vi "Display.vi"(8 "error in":errorcluster, 11 "Custom - One Button in":refnum<class "Custom - One Button.lvclass">) -> (0 "error out":errorcluster, 3 "Custom - One Button out":refnum<class "Custom - One Button.lvclass">)   [LabVIEW 2021, in "Pop-Up.lvlib" / "Custom - One Button.lvclass"]
doc: "This VI will display the custom image and message to the user\n\n<b>Code Developed By:</b> +\nDaniel Coons +\nhttps://github.com/danielcoons/tsc-pop-up"
uses:
  Custom - One Button.lvclass
  C:/Development/Open Source/tsc-pop-up/Popup/Popup.lvclass
  Popup/Popup.lvclass/Popup.ctl
  Popup/Data Member Access/Read Theme.vi
  Theme/Theme.lvclass
  Popup/Popup.lvclass
  user32.dll
panel:
  out "header":bool
  in  "OK":bool
  out "2D Picture":picture
  out "Message":string
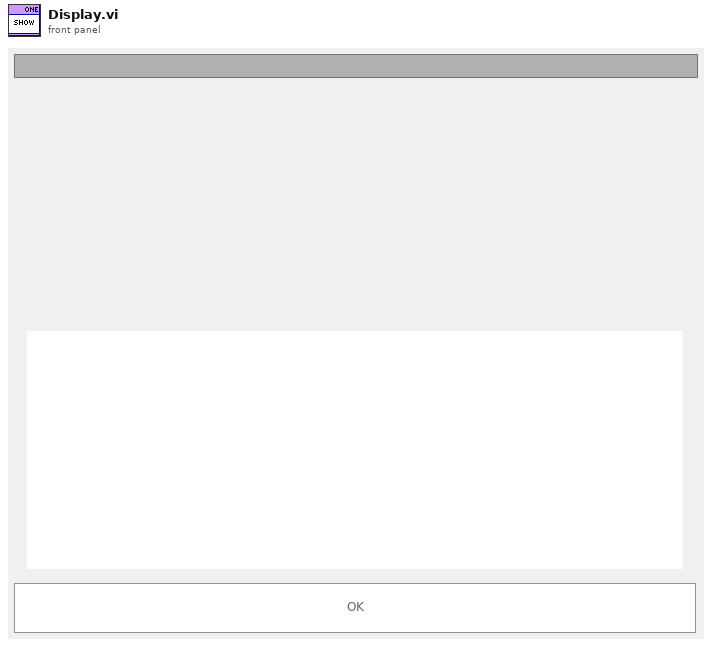
[diagram p1: front panel]
types:
  T1 = typedef "LVPoint32TypeDef.ctl" = cluster{"Horizontal":i32, "Vertical":i32}
  T2 = typedef "LVPositionTypeDef.ctl" = cluster{"Left":i32, "Top":i32}
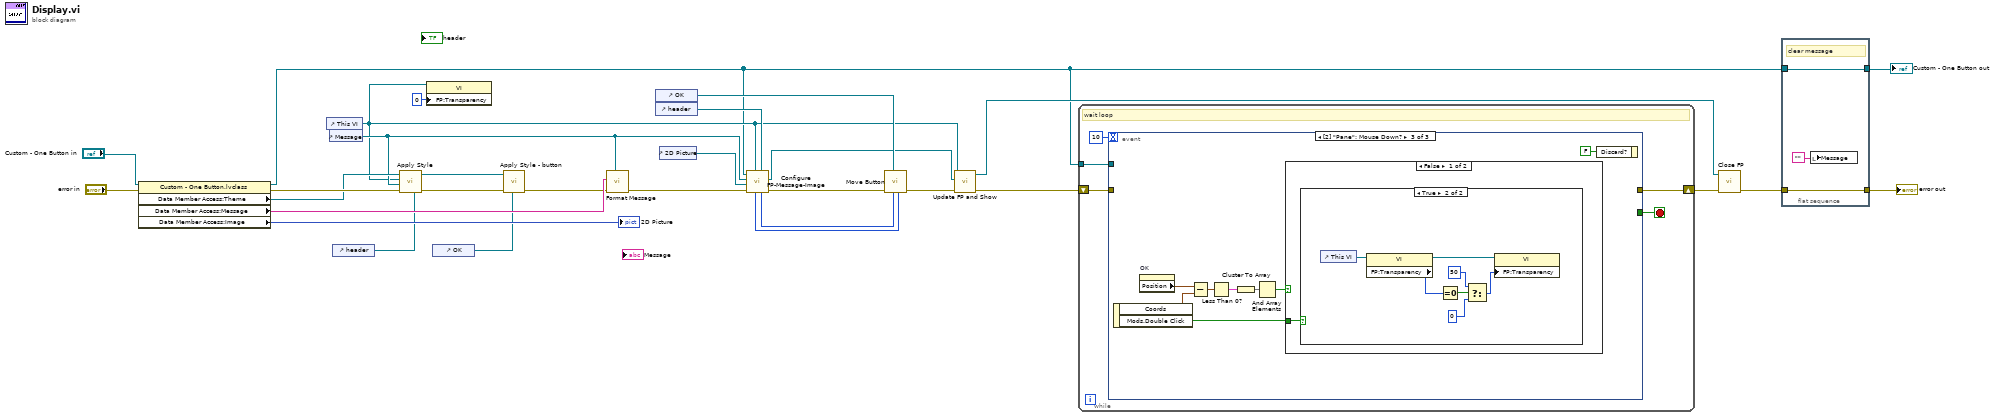
[diagram p0: block diagram]
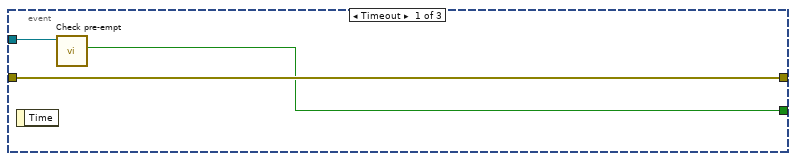
[diagram p2: hidden frame]
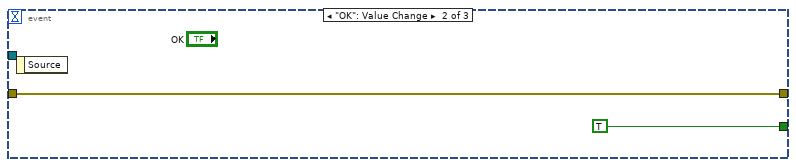
[diagram p3: hidden frame]
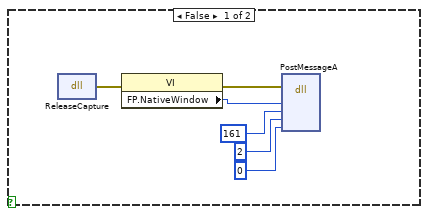
[diagram p4: hidden frame]
diagram:
  n1 = property class="Custom - One Button.lvclass"(reference="Custom - One Button in", error in="error in") -> (reference out=w1:refnum<class "Custom - One Button.lvclass">, error out=w26:errorcluster, "Data Member Access:Theme"=w21:refnum<class "Theme.lvclass">, "Data Member Access:Message"=w19:string, "Data Member Access:Image"=→"2D Picture":picture)
  n2 = control-ref of="This VI"() -> (w3:refnum<vi>)
  n3 = control-ref of="Message"() -> (w15:refnum<vi>)
  n4 = control-ref of="header"() -> (w7:refnum<vi>)
  n5 = call "Apply Style.vi"("header ref"=w7, "error in"=w26, "message ref"=w15, "pop up ref"=w3, "Theme in"=w21) -> ("error out"=w9:errorcluster, "Theme out"=w18:refnum<class "Theme.lvclass">)  [unwired: 5 in]
  n6 = property class="VI"(reference=w3, "FP:Transparency"=u8 0 ("Front Panel Window:Transparency")) -> ()  [unwired: 1 in, 2 out]
  n7 = control-ref of="OK"() -> (w17:refnum<vi>)
  n8 = call "Apply Style - button.vi"("button ref"=w17, "error in"=w9, "Theme in"=w18) -> ("error out"=w8:errorcluster)  [unwired: 7 in, 1 out]
  n9 = call "Format Message.vi"("formatted string"=w15, "error in"=w8, "String Input"=w19) -> ("error out"=w5:errorcluster)  [unwired: 7 in, 1 out]
  n10 = control-ref of="OK"() -> (w16:refnum<vi>)
  n11 = control-ref of="header"() -> (w10:refnum<vi>)
  n12 = control-ref of="2D Picture"() -> (w14:refnum<vi>)
  n13 = call "Configure FP-Message-Image.vi"("header ref"=w10, "Pop Up ref"=w3, "error in (no error)"=w5, "Image ref"=w14, "Message ref"=w15, "Popup in"=w1) -> ("error out"=w6:errorcluster, "Panel Ref"=w11:refnum<vi>, "Panel Width"=w13:i32, "Panel Height"=w12:i32)  [unwired: 1 in, 1 out]
  n14 = call "Move Button.vi"("Panel Height"=w12, "Panel Width"=w13, "Button"=w16, "error in"=w6) -> ("error out"=w25:errorcluster)  [unwired: 6 in, 1 out]
  n15 = call "Update FP and Show.vi"("error in (no error)"=w25, "Panel Ref"=w11, "VI in"=w3) -> ("error out"=w22:errorcluster, "VI out"=w4:refnum<vi>)  [unwired: 7 in]
  n16 = while {
    shift-right: [w35] -> w24
    shift-left: w22 -> [w34]
    tunnel: w1 -> [w31]
    stop <- w33 stop-if-true
    # "wait loop"
    n17 = event shown="[2] \"Pane\": Mouse Down?" {
      selector: _ -> [_ _ _]
      dyn-events: _ -> [_ _ _]
      timeout: 10 -> [_ _ _]
      tunnel: w34 -> [w38 w40 _]
      tunnel: [w38 w40 _] -> w35
      tunnel: [w36 TRUE _] -> w33
      tunnel: w31 -> [w37 _ _]
      event Timeout {
        n18 = event-data() -> ()  [unwired: 1 in, 1 out]
        n19 = call "Check pre-empt.vi"("_Popup in"=w37) -> ("Pre-empted?"=w36:bool)  [unwired: 8 in, 2 out]
      }
      event "OK": Value Change {
        n20 = event-data() -> ()  [unwired: 1 in, 1 out]
      }
      event Mouse Down? {
        n21 = event-data() -> ("Coords"=w41:T1, "Mods.Double Click"=w42:bool)  [unwired: 1 in]
        n22 = property on="OK" class="Bool"() -> ("Position"=w43:T2)  [unwired: 2 in, 2 out]
        n23 = Subtract(x=w43, y=w41) -> (x-y=w44:T2)
        n24 = Less Than 0?(x=w44) -> (x < 0?=w45:cluster{"Left":bool, "Top":bool})
        n25 = Cluster To Array(cluster=w45) -> (array=w46:bool[])
        n26 = And Array Elements(Boolean array=w46) -> (logical AND=w47:bool)
        n27 = case shown="False" w47 {
          tunnel: w42 -> [w49 _]
          frame False {
            n28 = case shown="True" w49 {
              frame False {
                n29 = dll-call lib="user32.dll" fn="ReleaseCapture"() -> (error out=w53:errorcluster)  [unwired: 4 in, 1 out]
                n30 = property class="VI"(error in=w53) -> (error out=w54:errorcluster, "FP.NativeWindow"=w55:u64)  [unwired: 1 in, 1 out]
                n31 = dll-call lib="user32.dll" fn="PostMessageA"(error in=w54, "hWnd"=w55, "Msg"=161, "wParam"=2, "lParam"=0) -> ()  [unwired: 7 in, 2 out]
              }
              frame True {
                n32 = control-ref of="This VI"() -> (w62:refnum<vi>)
                n33 = property class="VI"(reference=w62) -> (reference out=w60:refnum<vi>, "FP:Transparency"=w61:u8)  [unwired: 1 in, 1 out]
                n34 = Equal To 0?(x=w61) -> (x = 0?=w59:bool)
                n35 = Select(t=u8 50, s=w59, f=u8 0) -> (s? t:f=w58:u8)
                n36 = property class="VI"(reference=w60, "FP:Transparency"=w58) -> ()  [unwired: 1 in, 2 out]
              }
            }
          }
          frame True {
          }
        }
        n37 = event-data("Discard?"=FALSE) -> ()  [unwired: 1 in, 1 out]
      }
    }
  }
  n38 = call "Close FP.vi"("error in (no error)"=w24, "VI in"=w4) -> ("error out"=w23:errorcluster)  [unwired: 9 in]
  n39 = flat-sequence {
    tunnel: w23 -> [w65]
    tunnel: [w65] -> w27
    tunnel: w1 -> [w64]
    tunnel: [w64] -> w28
    frame #0 {
      # "clear message"
      n40 = local write "Message"("" ("Message")) -> ()
    }
  }
  "error out" <- w27
  "Custom - One Button out" <- w28
